vi "Get Pulse State.vi"(8 "error in (no error)":errorcluster, 11 "Pulse Recorder Actor in":refnum<class "Pulse Recorder Actor.lvclass">) -> (0 "error out":errorcluster, 1 "Result ready":bool, 2 "Armed":bool, 3 "Pulse Recorder Actor out":refnum<class "Pulse Recorder Actor.lvclass">)   [LabVIEW 2021, in "Pulse Recorder Actor.lvclass"]
uses:
  Pulse Recorder Actor.lvclass
  Read Pulse driver.vi
  Write Pulse driver.vi
  NHMFL_Core/Libraries/Instruments/Pulse Driver/Pulse Driver.lvclass
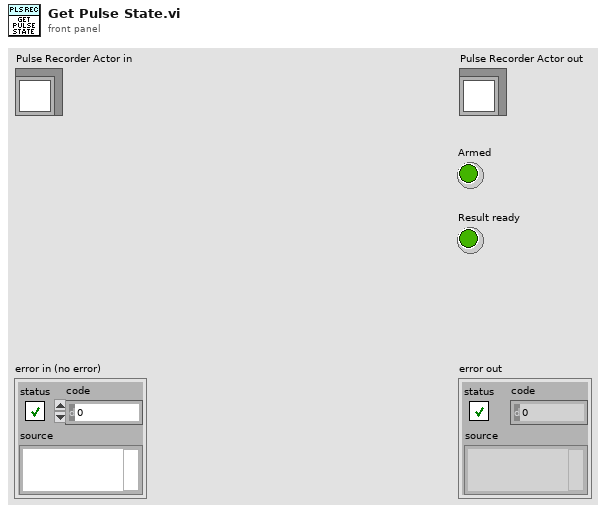
[diagram p1: front panel]
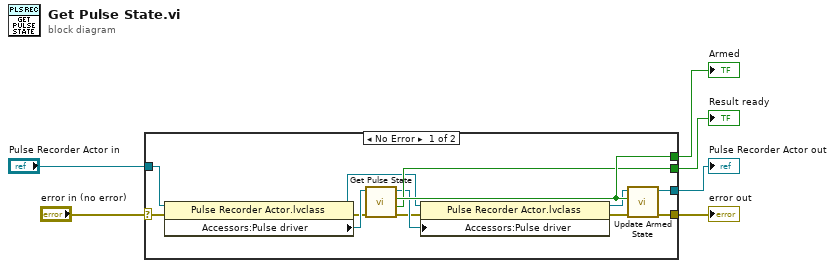
[diagram p0: block diagram]
diagram:
  n1 = case shown="No Error" "error in (no error)" {
    selector: "error in (no error)" -> [w17 w21]
    tunnel: [w19 w21] -> w2
    tunnel: [w18 w20] -> w1
    tunnel: "Pulse Recorder Actor in" -> [w11 w20]
    tunnel: [w14 _] -> w4
    tunnel: [w13 _] -> w3
    frame No Error {
      n2 = property class="Pulse Recorder Actor.lvclass"(reference=w11, error in=w17) -> (reference out=w7:refnum<class "Pulse Recorder Actor.lvclass">, error out=w15:errorcluster, "Accessors:Pulse driver"=w16:refnum<class "Pulse Driver.lvclass">)
      n3 = call-dynamic "Get Pulse State.vi"("error in (no error)"=w15, "Pulse Driver in"=w16) -> ("error out"=w9:errorcluster, "Result ready"=w13:bool, "Armed"=w14:bool, "Pulse Driver out"=w12:refnum<class "Pulse Driver.lvclass">)  [unwired: 5 in, 1 out]
      n4 = property class="Pulse Recorder Actor.lvclass"(reference=w7, error in=w9, "Accessors:Pulse driver"=w12) -> (reference out=w10:refnum<class "Pulse Recorder Actor.lvclass">, error out=w8:errorcluster)
      n5 = call-dynamic "Update Armed State.vi"("error in (no error)"=w8, "Armed"=w14, "Pulse Recorder in"=w10) -> ("error out"=w19:errorcluster, "Pulse Recorder out"=w18:refnum<class "Pulse Recorder Actor.lvclass">)  [unwired: 7 in]
    }
    frame Error {
    }
  }
  "error out" <- w2
  "Pulse Recorder Actor out" <- w1
  "Result ready" <- w3
  "Armed" <- w4
